vi "QueryFastRoutineResults.vi"(0 "System No.":i32=1, 1 "Fast Routine Names":string[](array[string]), 2 "No. Routines to query at once":i32=1, 5 "error in":errorcluster) -> (14 "Routine Results":T2(array[cluster]) {"Sys" min=1 step=1}, 19 "error out":errorcluster)   [LabVIEW 2014]
doc: "This VI queries FRR? and displays the results for the specified routines.\nThe parameters used for FRR? are 1, 2, 3 and 5.\nDue to limitations of the input buffer size for GCS commands at PI controllers, one can specify the number of Fast Alignment Routines to query with one FRR? command."
uses:
  C:/ProgramData/PI/LabVIEW/Low Level/General command.llb/Controller names.ctl
  C:/ProgramData/PI/LabVIEW/Low Level/General command.llb/Global2 (Array).vi
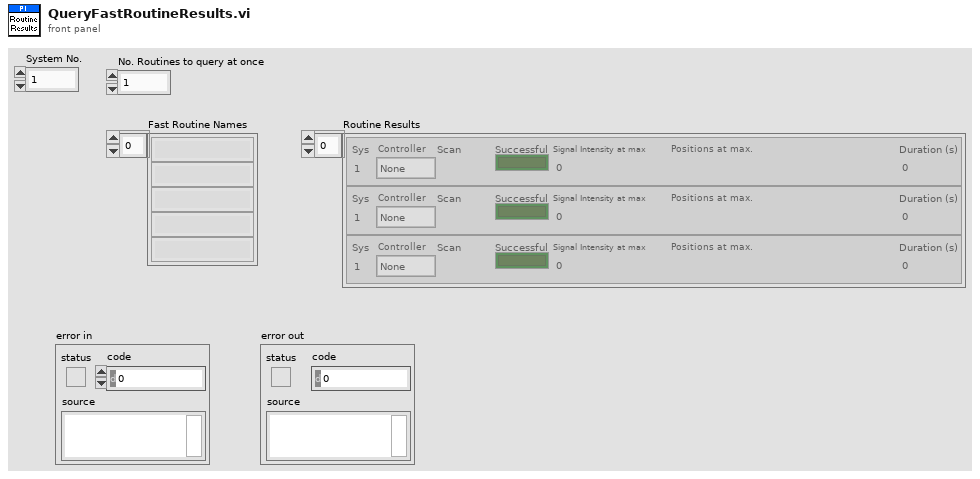
[diagram p1: front panel]
types:
  T1 = typedef "Controller names.ctl" = enum16{"None", "Analog", "C-702", "C-413", "C-414", "C-843", "C-843.PM", "C-844", "C-848", "C-865", "C-866", "C-867", "C-877", "C-880", "C-884", "C-885", "C-886", "C-887", "C-891", "E-135", "E-516", "E-517", "E-518", "E-709", "E-710", "E-712", "E-725", "E-727", "E-753", "E-754", "E-755", "E-761", "E-816", "E-861", "E-870", "E-871", "E-872", "E-873", "E-874", "F-206", "HydraPollux", "M-840", "M-850", "M-8X0", "Mercury", "Mercury_GCS", "PI_GCS2"}
  T2 = cluster{"Sys":i32, "Controller":T1, "Scan":string, "Successful":bool, "Signal Intensity at max":dbl, "Positions at max.":string, "Duration (s)":dbl}[]
  T3 = cluster{"System No.":i32, "Controller name":T1, "Scan Name":string, "Successful":bool, "Signal Intensity at max":dbl, "Positions at max.":string, "Duration (s)":dbl}[]
  T4 = cluster{"Conn. axes":string[], "Controller name":T1}[]
  T5 = cluster{"Conn. axes":string[], "Controller name":T1}
  T6 = cluster{"System No.":i32, "Controller":T1, "Scan Name":string, "Successful":bool, "Signal Intensity at max":dbl, "Positions at max.":string, "Duration (s)":dbl}
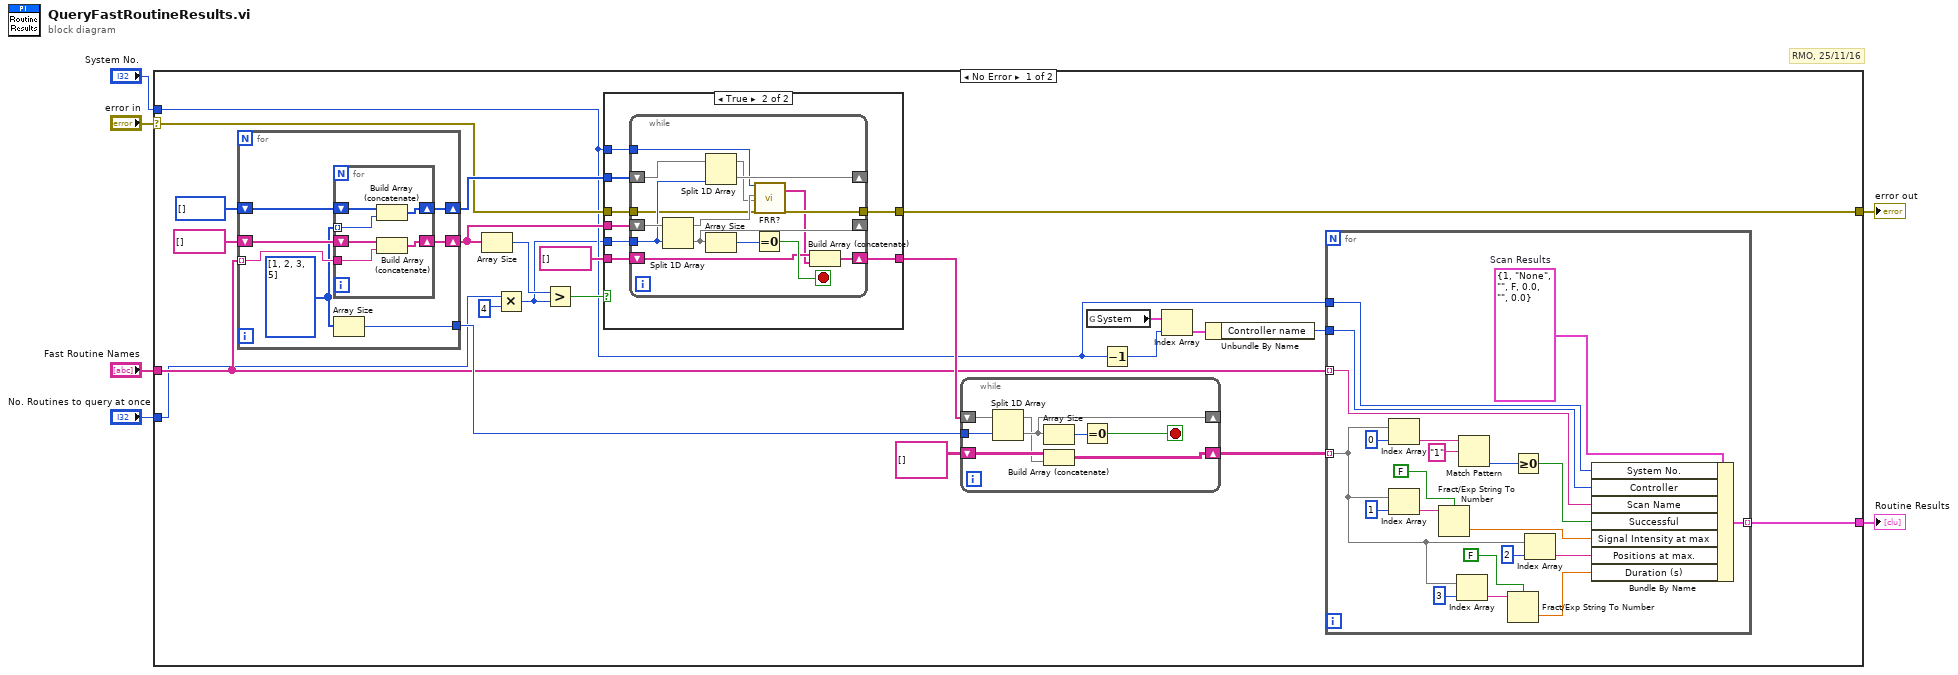
[diagram p0: block diagram]
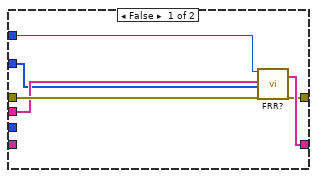
[diagram p2: hidden frame]
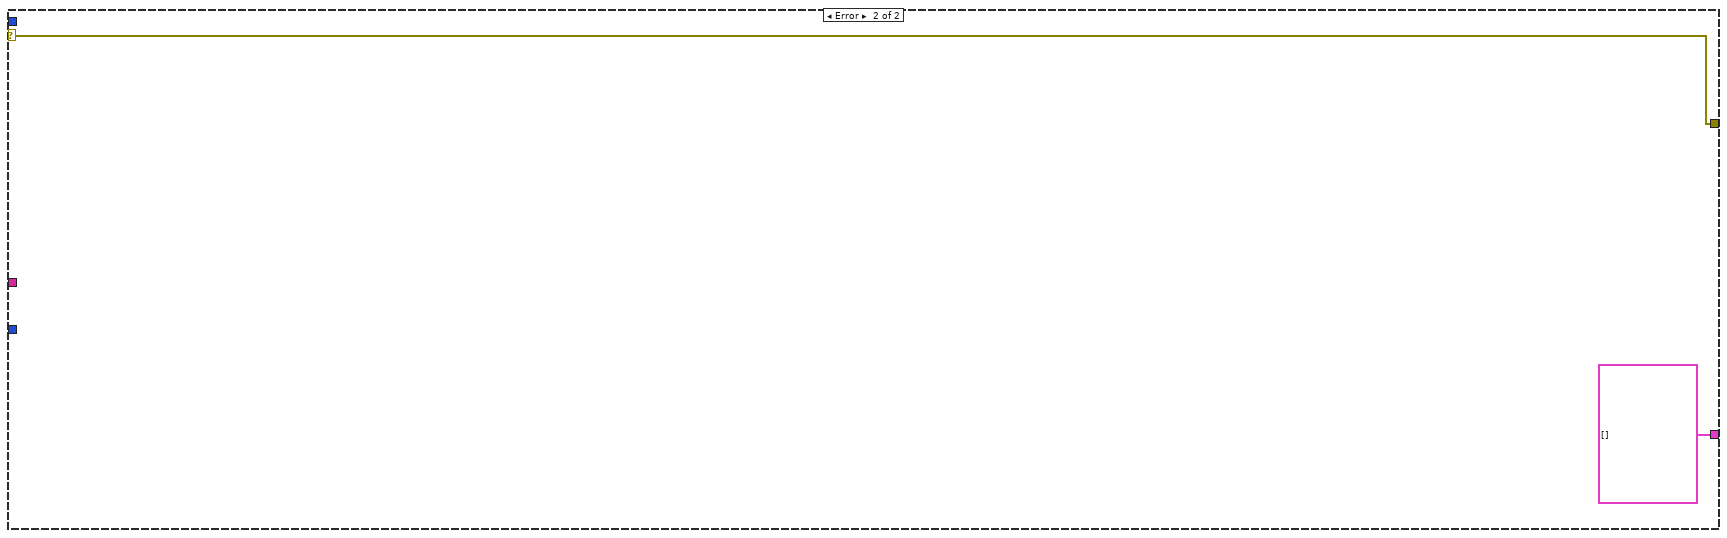
[diagram p3: hidden frame]
diagram:
  # "RMO, 25/11/16"
  n1 = case shown="No Error" "error in" {
    selector: "error in" -> [w18 w102]
    tunnel: "Fast Routine Names" -> [w10 _]
    tunnel: "System No." -> [w12 _]
    tunnel: [w16 w102] -> w3
    tunnel: [w24 T3 []] -> w2
    tunnel: "No. Routines to query at once" -> [w9 _]
    frame No Error {
      n2 = for {
        tunnel: w10 -> [w94] mode=indexing
        shift-right: [w90] -> w21
        shift-left: string[] [] -> [w93]
        shift-right: [w91] -> w20
        shift-left: i32[] [] -> [w92]
        tunnel: [w88] -> w26
        w89 = i32[] [1, 2, 3, 5] ("ResultID")
        n3 = for {
          tunnel: w89 -> [w96] mode=indexing
          tunnel: w94 -> [w99]
          shift-right: [w98] -> w90
          shift-left: w93 -> [w100]
          shift-right: [w95] -> w91
          shift-left: w92 -> [w97]
          n4 = Build Array (concatenate)(w97, w96) -> (w95:i32[])
          n5 = Build Array (concatenate)(w100, w99) -> (w98:string[])
        }
        n6 = Array Size(array=w89) -> (size(s)=w88:i32)
      }
      n7 = Array Size(array=w21) -> (size(s)=w23:i32)
      n8 = Multiply(x=w9, y=4) -> (x*y=w7:i32)
      n9 = Greater?(x=w23, y=w7) -> (0:w22:bool)
      n10 = case shown="True" w22 {
        tunnel: w21 -> [w33 w43]
        tunnel: w7 -> [_ w42]
        tunnel: w20 -> [w32 w41]
        tunnel: string[] [] -> [_ w40]
        tunnel: w12 -> [w35 w39]
        tunnel: w18 -> [w34 w38]
        tunnel: [w30 w37] -> w16
        tunnel: [w31 w36] -> w17
        frame False {
          n11 = call "FRR?.vi"("System no."=w35, "Routinename"=w33, "ResultID"=w32, "error in"=w34) -> ("Value (string)"=w31:string[], "error out"=w30:errorcluster)  [unwired: 2 in, 12 out]
        }
        frame True {
          n12 = while {
            shift-right: [w57] -> _
            shift-left: w43 -> [w58]
            tunnel: w42 -> [w52]
            shift-right: [w53] -> _
            shift-left: w41 -> [w54]
            shift-right: [w44] -> w36
            shift-left: w40 -> [w46]
            tunnel: w39 -> [w51]
            tunnel: w38 -> [w48]
            tunnel: [w47] -> w37
            stop <- w55 stop-if-true
            n13 = Split 1D Array(array=w58, index=w52) -> (first subarray=w50:string[], second subarray=w57:string[])
            n14 = Split 1D Array(array=w54, index=w52) -> (first subarray=w49:i32[], second subarray=w53:i32[])
            n15 = Array Size(array=w57) -> (size(s)=w56:i32)
            n16 = Equal To 0?(x=w56) -> (x = 0?=w55:bool)
            n17 = call "FRR?.vi"("System no."=w51, "Routinename"=w50, "ResultID"=w49, "error in"=w48) -> ("Value (string)"=w45:string[], "error out"=w47:errorcluster)  [unwired: 2 in, 12 out]
            n18 = Build Array (concatenate)(w46, w45) -> (w44:string[])
          }
        }
      }
      n19 = while {
        shift-right: [w84] -> _
        shift-left: w17 -> [w87]
        shift-right: [w85] -> w25
        shift-left: string[][] [] -> [w86]
        tunnel: w26 -> [w81]
        stop <- w82 stop-if-true
        n20 = Split 1D Array(array=w87, index=w81) -> (first subarray=w80:string[], second subarray=w84:string[])
        n21 = Array Size(array=w84) -> (size(s)=w83:i32)
        n22 = Build Array (concatenate)(w86, w80) -> (w85:string[][])
        n23 = Equal To 0?(x=w83) -> (x = 0?=w82:bool)
      }
      n24 = global read "Global2 (Array).vi" "System"() -> (w15:T4)
      n25 = Decrement(x=w12) -> (x-1=w14:i32)
      n26 = Index Array(array=w15, index=w14) -> (element=w13:T5)
      n27 = Unbundle By Name(w13) -> ("Controller name"=w11:T1)
      n28 = for {
        tunnel: w25 -> [w79] mode=indexing
        tunnel: [w66] -> w24 mode=indexing
        tunnel: w12 -> [w61]
        tunnel: w11 -> [w60]
        tunnel: w10 -> [w59] mode=indexing
        w70 = T6 {"System No."=1, "Controller"=enum."None", "Scan Name"="", "Successful"=FALSE, "Signal Intensity at max"=0.0, "Positions at max."="", "Duration (s)"=0.0}  # Scan Results
        n29 = Index Array(array=w79, index=0) -> (element=w65:string)
        n30 = Index Array(array=w79, index=1) -> (element=w75:string)
        n31 = Fract/Exp String To Number(use system decimal point (T)=FALSE, string=w75) -> (number=w69:dbl)  [unwired: 3 out]
        n32 = Index Array(array=w79, index=3) -> (element=w72:string)
        n33 = Match Pattern(string=w65, regular expression="1") -> (offset past match=w63:i32)  [unwired: 4 out]
        n34 = Fract/Exp String To Number(use system decimal point (T)=FALSE, string=w72) -> (number=w67:dbl)  [unwired: 3 out]
        n35 = Greater Or Equal To 0?(x=w63) -> (x >= 0?=w62:bool)
        n36 = Index Array(array=w79, index=2) -> (element=w68:string)
        n37 = Bundle By Name(cluster=w70, "System No."=w61, "Controller"=w60, "Scan Name"=w59, "Successful"=w62, "Signal Intensity at max"=w69, "Positions at max."=w68, "Duration (s)"=w67) -> (w66:T6)
      }
    }
    frame Error {
    }
  }
  "error out" <- w3
  "Routine Results" <- w2
